vi "StoreResult.vi"(8 "error in (no error)":errorcluster, 10 "Table name":string="TestResult", 11 "区域管理":T1) -> (0 "error out":errorcluster={"status"=TRUE, "code"=1, "source"="DB Tools Validate Inputs.vi->DB Tools Insert Data.vi->StoreUUTResult.vi<ERR>Argument error. The table name given is blank."})   [LabVIEW 2014, in "DataBase.lvlib"]
uses:
  DataBase.lvlib
  <vilib>/addons/database/Connection.llb/DB Tools Open Connec (String).vi
  <vilib>/addons/database/NI_Database_API.lvlib
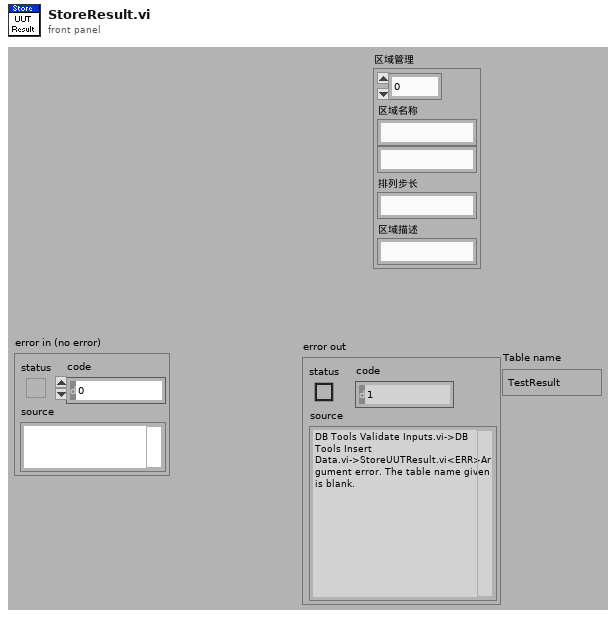
[diagram p1: front panel]
types:
  T1 = cluster{i32, "区域名称":string, string, "排列步长":string, "区域描述":string}
  T2 = typedef "NI_Database_API.lvlib/Conn ObjectReference.ctl" = refnum<k1>
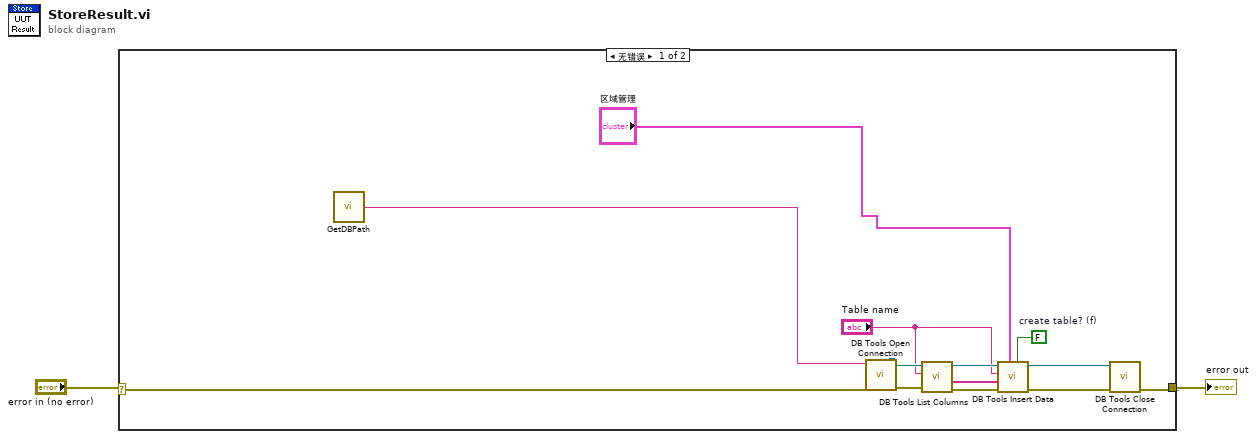
[diagram p0: block diagram]
diagram:
  n1 = case shown="无错误" "error in (no error)" {
    selector: "error in (no error)" -> [w13 w16]
    tunnel: [w12 w16] -> w1
    frame No Error {
      w11 = FALSE  # create table? (f)
      n2 = call "GetDBPath.vi"() -> ("Connection"=w4:string)  [unwired: 1 in]
      n3 = call-poly <vilib>:"DB Tools Open Connection.vi"("error in (no error)"=w13, "connection information"=w4) -> ("error out"=w9:errorcluster, "connection reference"=w10:T2)  [unwired: 6 in]
      n4 = call <vilib>:"DB Tools List Columns.vi"("error in (no error)"=w9, "table"="Table name", "connection reference"=w10) -> ("error out"=w7:errorcluster, "columns"=w6:string[], "connection reference out"=w8:T2)  [unwired: 1 in, 1 out]
      n5 = call <vilib>:"DB Tools Insert Data.vi"("create table? (F)"=w11, "data"="区域管理", "error in (no error)"=w7, "columns"=w6, "table"="Table name", "connection reference"=w8) -> ("error out"=w14:errorcluster, "connection reference out"=w15:T2)  [unwired: 4 in]
      n6 = call <vilib>:"DB Tools Close Connection.vi"("error in (no error)"=w14, "connection reference"=w15) -> ("error out"=w12:errorcluster)  [unwired: 5 in]
    }
    frame Error {
    }
  }
  "error out" <- w1
